vi "Set GPU View.vi"(8 "error in (no error)":errorcluster, 10 "GPU View":T1 {"fwidth:" format="%#_6p"; "f0:" format="%#_6p"}, 11 "Application Manager in":refnum<class "Application Manager.lvclass">) -> (0 "error out":errorcluster, 3 "Application Manager out":refnum<class "Application Manager.lvclass">)   [LabVIEW 2020, in "Application Manager.lvlib" / "Application Manager.lvclass"]
uses:
  Application Manager.lvclass
  chart zoom.ctl
  Application Manager.lvclass/Application Manager.ctl
  GPU FFT Calculator/GPU FFT Calculator Messages/Write GPU View Msg/Write GPU View Msg.lvclass/Write GPU View Msg.ctl
  <vilib>/ActorFramework/Message Enqueuer/Message Enqueuer.lvclass/Message Enqueuer.ctl
  <vilib>/ActorFramework/Message Enqueuer/Enqueue.vi
  GPU FFT Calculator/GPU FFT Calculator Messages/Write GPU View Msg/Write GPU View Msg.lvclass
  C:/Program Files/National Instruments/LabVIEW 2026/vi.lib/ActorFramework/Message/Message.lvclass
  <vilib>/ActorFramework/Message Priority Queue/Priority Enqueue.vi
  Simple UI/Simple UI/Simple UI.lvclass
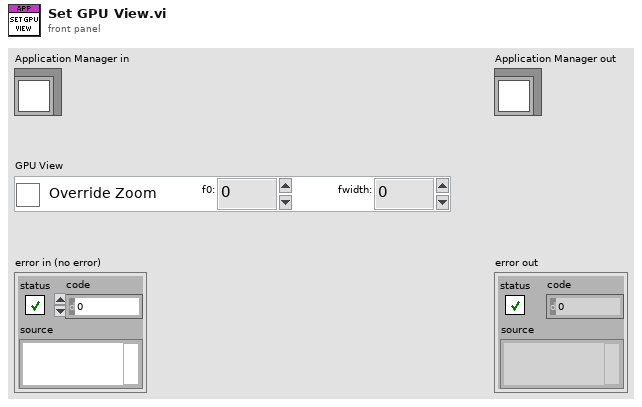
[diagram p1: front panel]
types:
  T1 = typedef "Simple UI.lvlib/Simple UI.lvclass/chart zoom.ctl" = cluster{"Override":bool, "f0: ":dbl, "fwidth: ":dbl}
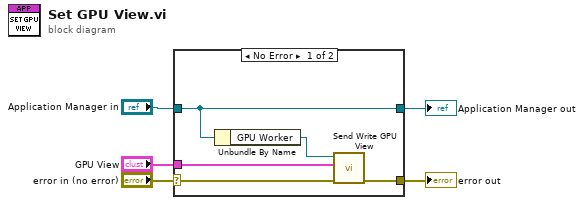
[diagram p0: block diagram]
diagram:
  n1 = case shown="No Error" "error in (no error)" {
    selector: "error in (no error)" -> [w7 w12]
    tunnel: [w6 w12] -> w4
    tunnel: [w10 w11] -> w2
    tunnel: "Application Manager in" -> [w10 w11]
    tunnel: "GPU View" -> [w8 _]
    frame No Error {
      n2 = Unbundle By Name(w10) -> ("GPU Worker"=w9:refnum<class "Message Enqueuer.lvclass">)
      n3 = call "Send Write GPU View.vi"("error in (no error)"=w7, "Cluster"=w8, "Message Enqueuer"=w9) -> ("error out"=w6:errorcluster)  [unwired: 7 in, 1 out]
    }
    frame Error {
    }
  }
  "error out" <- w4
  "Application Manager out" <- w2
